vi "str2bitmap.vi"(8 "error in":errorcluster, 10 "file":path=path "C:/Users/yaroslav/Desktop/st7558_i2c/font.bin", 11 "String":string) -> (0 "error out":errorcluster, 3 "bitmap":u8[](array[numeric]) format="%x")   [LabVIEW 2017]
panel:
  out "ASCII position":u8[](array[numeric])
  out "font_array":u8[](array[numeric]) format="%x"
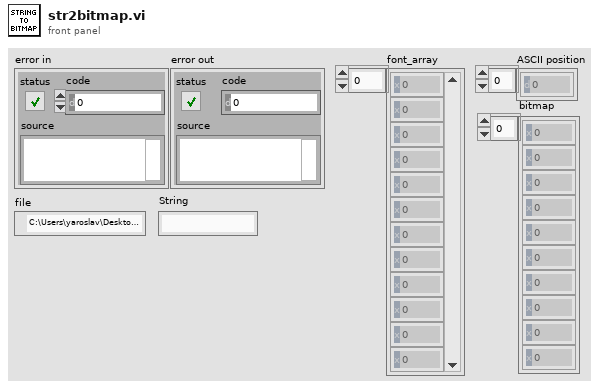
[diagram p1: front panel]
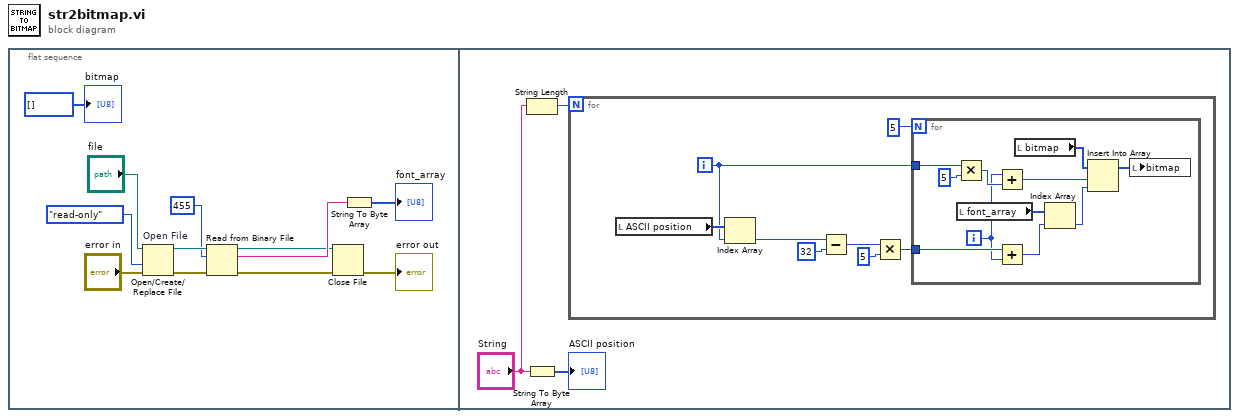
[diagram p0: block diagram]
diagram:
  n1 = flat-sequence {
    frame #0 {
      n2 = Open/Create/Replace File "Open File"(file path (use dialog)="file", error in="error in", access (0:read/write)=enum16{"read/write", "read-only", "write-only"}."read-only") -> (refnum out=w12:refnum<file>, error out=w5:errorcluster)  [unwired: 3 in, 1 out]
      n3 = Read from Binary File(8:w5, 10:455 ("count (1)"), 11:w12) -> (0:w2:errorcluster, 2:w10:string, 3:w4:refnum<file>)  [unwired: 3 in, 1 out]
      n4 = Close File(refnum=w4, error in=w2) -> (error out=→"error out":errorcluster)  [unwired: 1 out]
      n5 = String To Byte Array(string=w10) -> (unsigned byte array=→"font_array":u8[])
      "bitmap" <- u8[] []
    }
    frame #1 {
      n6 = String Length(string="String") -> (length=w15:i32)
      n7 = String To Byte Array(string="String") -> (unsigned byte array=→"ASCII position":u8[])
      n8 = for {
        N: w15 -> [_]
        i -> [w16]
        n9 = local read "ASCII position"() -> (w23:u8[])
        n10 = Index Array "Index Array"(array=w23, index=w16) -> (element=w22:u8)
        n11 = Subtract(x=w22, y=32) -> (x-y=w20:i32)
        n12 = Multiply(x=w20, y=5) -> (x*y=w18:i32)
        n13 = for {
          N: 5 -> [_]
          tunnel: w18 -> [w34]
          tunnel: w16 -> [w31]
          i -> [w26]
          n14 = Multiply(x=w31, y=5) -> (x*y=w29:i32)
          n15 = local read "font_array"() -> (w33:u8[])
          n16 = Add(x=w26, y=w29) -> (x+y=w25:i32)
          n17 = Add(x=w34, y=w26) -> (x+y=w32:i32)
          n18 = local read "bitmap"() -> (w27:u8[])
          n19 = Index Array "Index Array"(array=w33, index=w32) -> (element=w24:u8)
          n20 = Insert Into Array "Insert Into Array"(array=w27, index=w25, new element=w24) -> (w28:u8[])
          n21 = local write "bitmap"(w28) -> ()
        }
      }
    }
  }
